vi "defer panel updates Controlref step1.vi"(8 "error in (no error)":errorcluster, 11 "control reference":refnum<vi>) -> (0 "error out":errorcluster, 3 "Refs":T1)   [LabVIEW 2020, in "Defer Panel Updates OpenSource.lvlib"]
doc: "This VI will defer front panel updates for the input control reference.\n\nWire the output of this VI to Step #2 to turn off deferment"
uses:
  Defer Panel Updates OpenSource.lvlib
  defer panel updates data.ctl
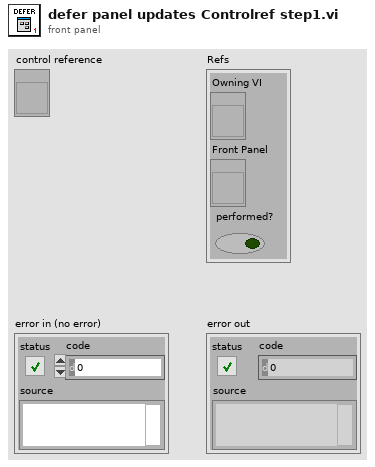
[diagram p1: front panel]
types:
  T1 = typedef "Defer Panel Updates OpenSource.lvlib/defer panel updates data.ctl" = cluster{"Owning VI":refnum<vi>, "Front Panel":refnum<vi>, "performed?":bool}
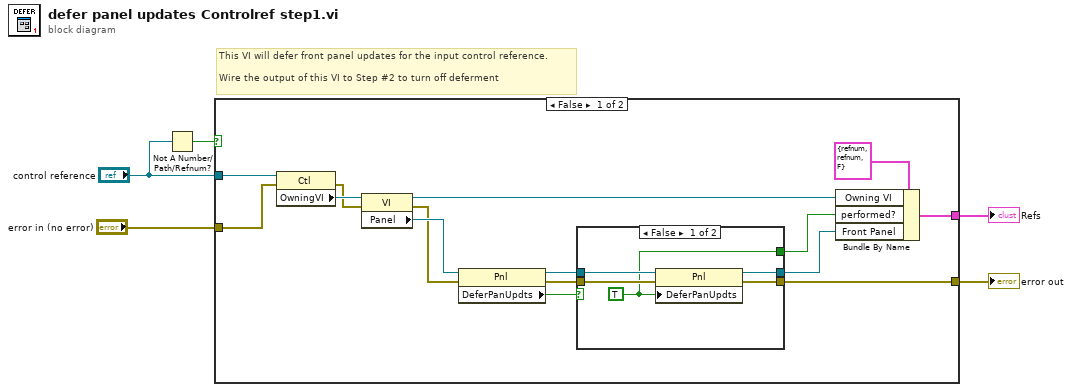
[diagram p0: block diagram]
diagram:
  # "This VI will defer front panel updates for the input control reference.\n\nWire the output of this VI to Step #2 to turn off deferment"
  n1 = Not A Number/Path/Refnum?(number/path/refnum="control reference") -> (NaN/Path/Refnum?=w5:bool)
  n2 = case shown="False" w5 {
    tunnel: "control reference" -> [w20 _]
    tunnel: "error in (no error)" -> [w15 w28]
    tunnel: [w13 w28] -> w2
    tunnel: [w12 _] -> w1
    frame False {
      n3 = property class="Ctl"(reference=w20, error in=w15) -> (error out=w14:errorcluster, "OwningVI"=w19:refnum<vi>)  [unwired: 1 out]
      n4 = property class="VI"(reference=w19, error in=w14) -> (reference out=w17:refnum<vi>, error out=w10:errorcluster, "Panel"=w11:refnum<vi>)
      n5 = property class="Pnl"(reference=w11, error in=w10) -> (reference out=w8:refnum<vi>, error out=w9:errorcluster, "DeferPanUpdts"=w7:bool)
      n6 = case shown="False" w7 {
        tunnel: [w25 w27] -> w16
        tunnel: [w24 w26] -> w13
        tunnel: w9 -> [w23 w26]
        tunnel: w8 -> [w22 w27]
        tunnel: [w21 _] -> w6
        frame False {
          w21 = TRUE ("Defer Panel Updates")
          n7 = property class="Pnl"(reference=w22, error in=w23, "DeferPanUpdts"=w21) -> (reference out=w25:refnum<vi>, error out=w24:errorcluster)
        }
        frame True {
        }
      }
      n8 = Bundle By Name(cluster=T1 {"Owning VI"=refnum, "Front Panel"=refnum, "performed?"=FALSE}, "Owning VI"=w17, "performed?"=w6, "Front Panel"=w16) -> (w12:T1)
    }
    frame True {
    }
  }
  "error out" <- w2
  "Refs" <- w1
